vi "CanInstallUninstall.vi"(6 "Auto-select Dependencies (T)":bool=TRUE, 7 "Version Selection (Highest)":u32[](array[ring]) items=["Highest", "Exactly"], 8 "error in (no error)":errorcluster, 9 "Software to Install":T1[](array[typedef]) {"component type" items=["standard", "hidden", "system", "unknown", "startup", "image"]}, 10 "Software to Uninstall":string[](array[string]), 11 "Session in":refnum<k21>) -> (0 "error out":errorcluster, 1 "Broken Dependencies":T3[](array[typedef]) {"dependee"."component type" items=["standard", "hidden", "system", "unknown", "startup", "image"]; "depender"."component type" items=["standard", "hidden", "system", "unknown", "startup", "image"]}, 3 "Session out":refnum<k21>)   [LabVIEW 2014, in "nisyscfg.lvlib"]
uses:
  nisyscfg.lvlib
  Broken Dependency 1.2.ctl
  Software 1.2.ctl
  Component Type.ctl
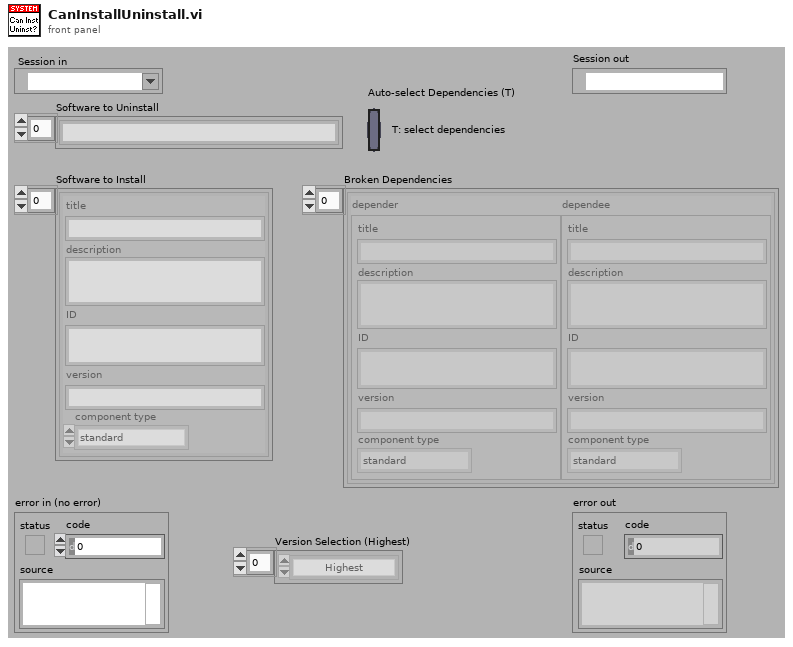
[diagram p1: front panel]
types:
  T1 = typedef "nisyscfg.lvlib/Software 1.2.ctl" = cluster{"title":string, "description":string, "ID":string, "version":string, "component type":T2}
  T2 = typedef "nisyscfg.lvlib/Component Type.ctl" = u32
  T3 = typedef "nisyscfg.lvlib/Broken Dependency 1.2.ctl" = cluster{"depender":T1, "dependee":T1}
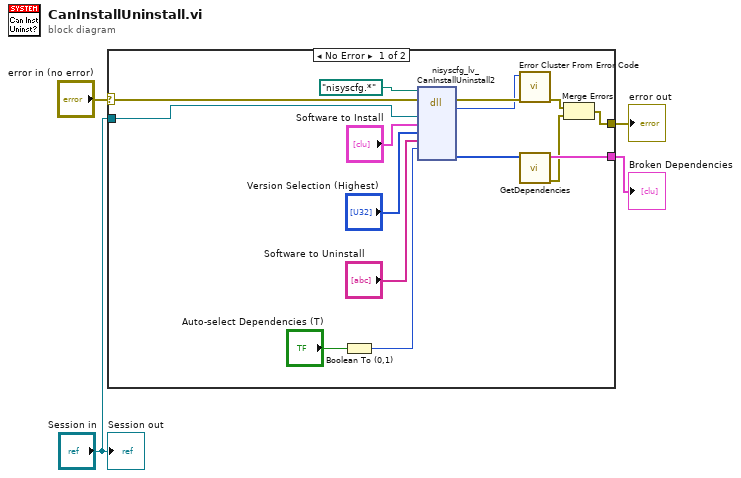
[diagram p0: block diagram]
diagram:
  n1 = case shown="No Error" "error in (no error)" {
    selector: "error in (no error)" -> [w11 w20]
    tunnel: "Session in" -> [w10 _]
    tunnel: [w5 w20] -> w3
    tunnel: [w12 _] -> w2
    frame No Error {
      n2 = Boolean To (0,1)(Boolean="Auto-select Dependencies (T)") -> (0, 1=w14:i16)
      n3 = dll-call lib="nisyscfg.*" fn="nisyscfg_lv_CanInstallUninstall2" label="CanInstallUninstall"(path in=path "nisyscfg.*", error in=w11, "session"=w10, "softwareToInstall"="Software to Install", "versionSelectionModes"="Version Selection (Highest)", "softwareIDsToUninstall"="Software to Uninstall", "autoSelectDependencies"=w14) -> (error out=w19:errorcluster, "result"=w18:i32, "brokenDependencies"=w13:u64[])  [unwired: 7 in, 1 out]
      n4 = call "Error Cluster From Error Code.vi"("error in (no error)"=w19, "error code (0)"=w18) -> ("error out"=w6:errorcluster)  [unwired: 7 in]
      n5 = call "GetDependencies.vi"("Enumerator in"=w13) -> ("error out"=w7:errorcluster, "Dependencies"=w12:T3[])  [unwired: 9 in]
      n6 = Merge Errors(w6, w7) -> (w5:errorcluster)
    }
    frame Error {
    }
  }
  "error out" <- w3
  "Broken Dependencies" <- w2
  "Session out" <- "Session in"
